vi "CommLoadDataNoteBegin.vi"(8 "error in (no error)":errorcluster, 10 "XML Refnum in":refnum<file>, 11 "Parameters In":refnum<class "Parameters.lvclass">) -> (0 "error out":errorcluster, 2 "XML Refnum out":refnum<file>, 3 "Parameters Out":refnum<class "Parameters.lvclass">)   [LabVIEW 2013, in "Parameters.lvclass"]
uses:
  Parameters.lvclass
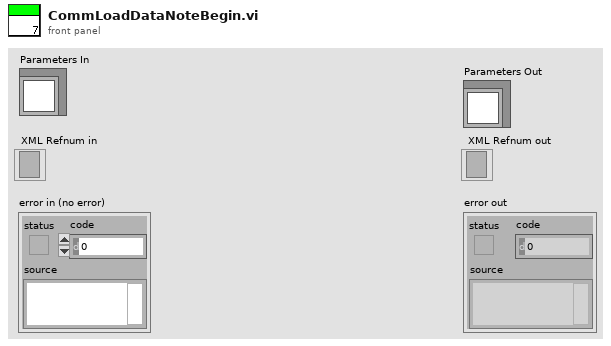
[diagram p1: front panel]
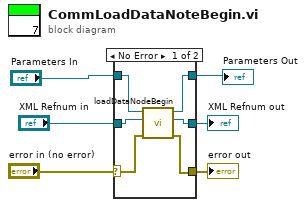
[diagram p0: block diagram]
diagram:
  n1 = case shown="No Error" "error in (no error)" {
    selector: "error in (no error)" -> [w10 w15]
    tunnel: [w9 w15] -> w5
    tunnel: [w7 w14] -> w1
    tunnel: "Parameters In" -> [w12 w14]
    tunnel: [w8 w13] -> w4
    tunnel: "XML Refnum in" -> [w11 w13]
    frame No Error {
      n2 = call-dynamic "loadDataNodeBegin.vi"("error in (no error)"=w10, "XML Refnum in"=w11, "Parameters in"=w12) -> ("error out"=w9:errorcluster, "XML Refnum out"=w8:refnum<file>, "Parameters out"=w7:refnum<class "Parameters.lvclass">)  [unwired: 6 in]
    }
    frame Error {
    }
  }
  "error out" <- w5
  "XML Refnum out" <- w4
  "Parameters Out" <- w1
